vi "get_virtual_folder_reference.vi"(7 "error in (no error)":errorcluster, 9 "name of virtual folder":string="accessors", 10 "new class reference in":refnum<vi>) -> (0 "error out":errorcluster, 3 "virtual folder ref out":refnum<vi>)   [LabVIEW 2010]
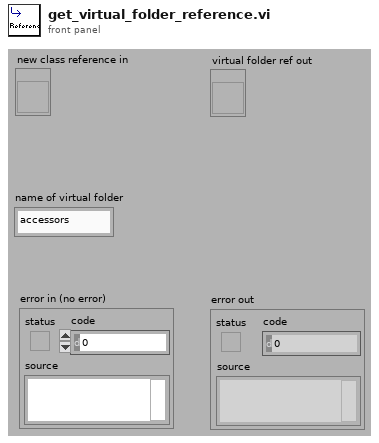
[diagram p1: front panel]
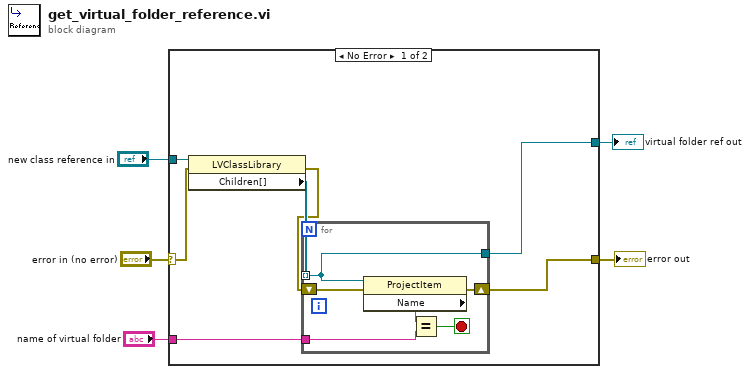
[diagram p0: block diagram]
diagram:
  n1 = case shown="No Error" "error in (no error)" {
    selector: "error in (no error)" -> [w11 w20]
    tunnel: "new class reference in" -> [w12 w19]
    tunnel: [w6 w19] -> w4
    tunnel: [w10 w20] -> w2
    tunnel: "name of virtual folder" -> [w7 _]
    frame No Error {
      n2 = property class="LVClassLibrary"(reference=w12, error in=w11) -> (error out=w8:errorcluster, "Children[]"=w9:refnum<vi>[])  [unwired: 1 out]
      n3 = for {
        tunnel: w9 -> [w16] mode=indexing
        shift-right: [w18] -> w10
        shift-left: w8 -> [w17]
        tunnel: w7 -> [w13]
        tunnel: [w16] -> w6
        stop <- w15 stop-if-true
        n4 = property class="ProjectItem"(reference=w16, error in=w17) -> (error out=w18:errorcluster, "Name"=w14:string)  [unwired: 1 out]
        n5 = Equal?(x=w14, y=w13) -> (x = y?=w15:bool)
      }
    }
    frame Error {
    }
  }
  "virtual folder ref out" <- w4
  "error out" <- w2
